vi "test.vi"() -> ()   [LabVIEW 2010, in "FPGAWrapperAK101022Resonance.lvclass"]
uses:
  FPGAWrapperAK101022Resonance.lvclass
  scan_specification_cluster.ctl
  class_data.vi
  Program Files (x86)/National Instruments/LabVIEW 2010/resource/objmgr/ni.dex.rc
panel:
  in  "sine mode?":bool
  out "Intensity output":i16[](graph)
  in  "Intensity amplitude":dbl
  out "channelA 2D":dbl[][](graph)
  out "channelA":dbl[](array[numeric])
  out "Available Elements for Reading":i32
  out "DAQ loop error out":errorcluster
  out "FPGA_AK101022Resonance out":refnum<class "FPGAWrapperAK101022Resonance.lvclass">
  in  "scan specification":T1
  in  "number of channels":i32=2
  in  "block size":i32=10000
  out "channel data block":dbl[][](graph)
  in  "timeout (ms)":i32=500
  out "timed out?":bool
  out "DAQ loop counter":i32=9010145
  in  "run button":bool
  in  "stop":bool
  # "Test VI for FGPA_AK101022Resonance"
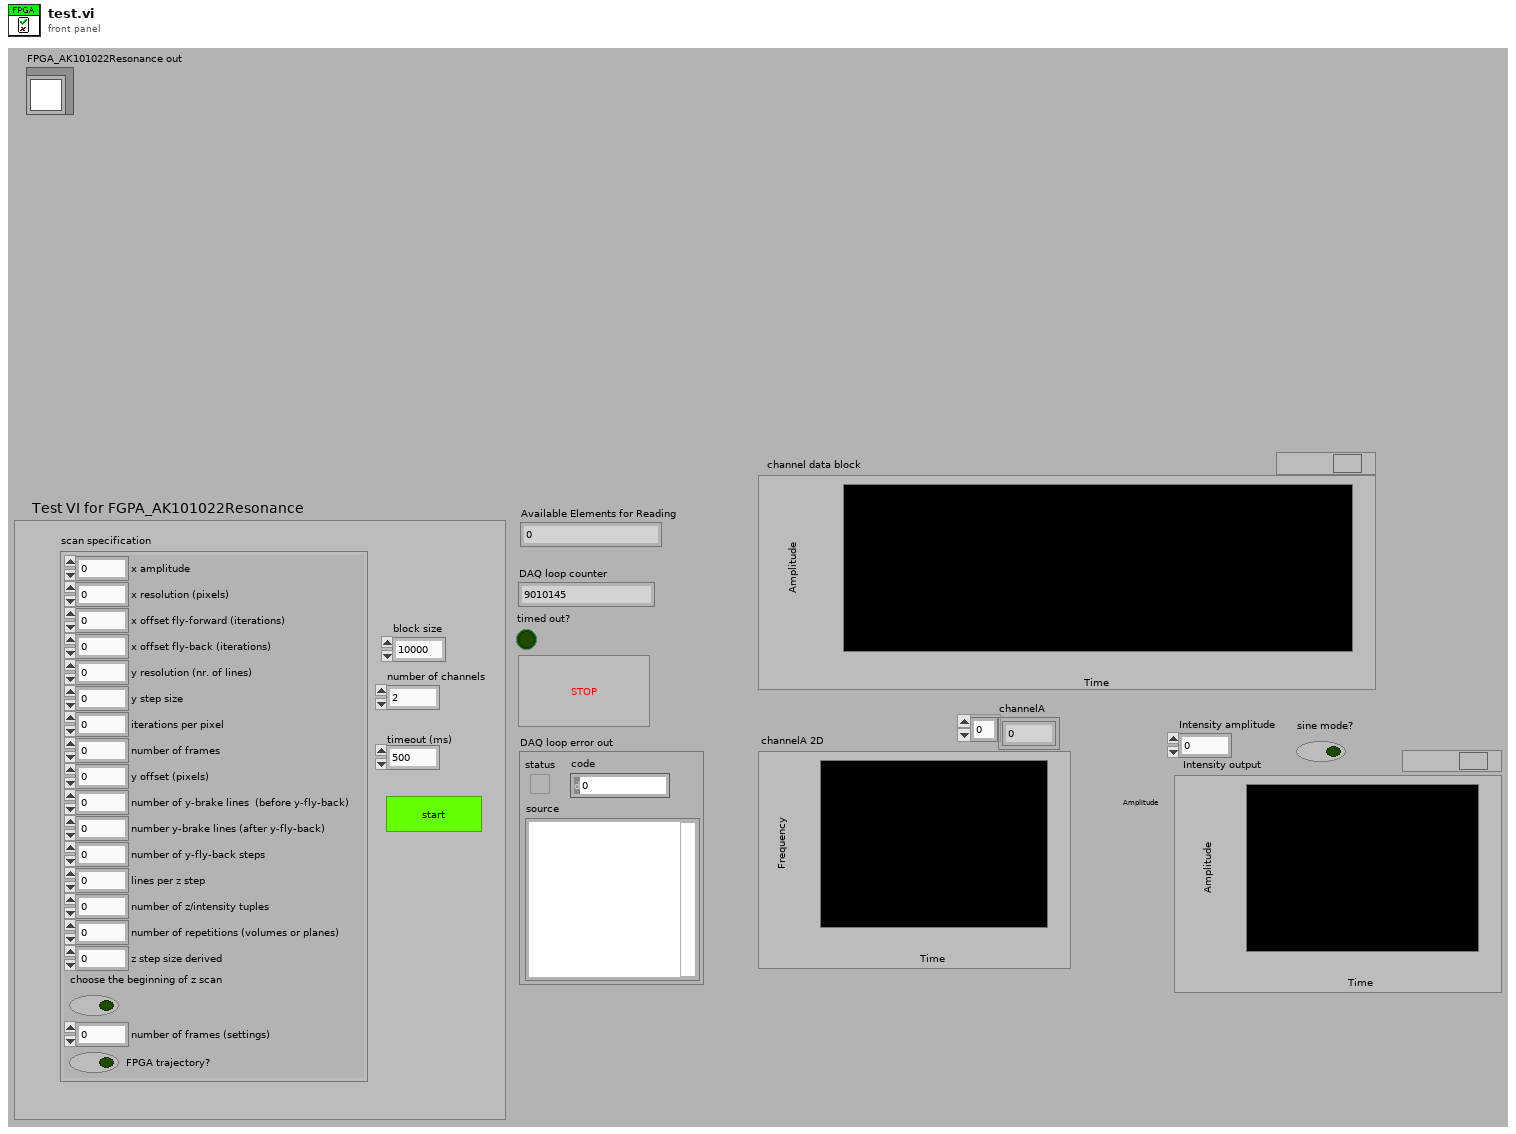
[diagram p1: front panel]
types:
  T1 = typedef "scan_specification_cluster.ctl" = cluster{"x amplitude":u16, "x resolution (pixels)":u16, "x offset fly-forward (iterations)":u16, "x offset fly-back (iterations)":u16, "y resolution (nr. of lines)":u16, "y step size":u16, "iterations per pixel":u16, "number of frames":i32, "y offset (pixels)":u16, "number of y-brake lines  (before y-fly-back)":u16, "number y-brake lines (after y-fly-back)":u16, "number of y-fly-back steps":u16, "lines per z step":u16, "number of z/intensity tuples":u16, "number of repetitions (volumes or planes)":i32, "z step size derived":u16, "choose the beginning of z scan":bool, "number of frames (settings)":i32, "FPGA trajectory?":bool}
  T2 = typedef "pixel_raw_data_array.ctl" = dbl[][]
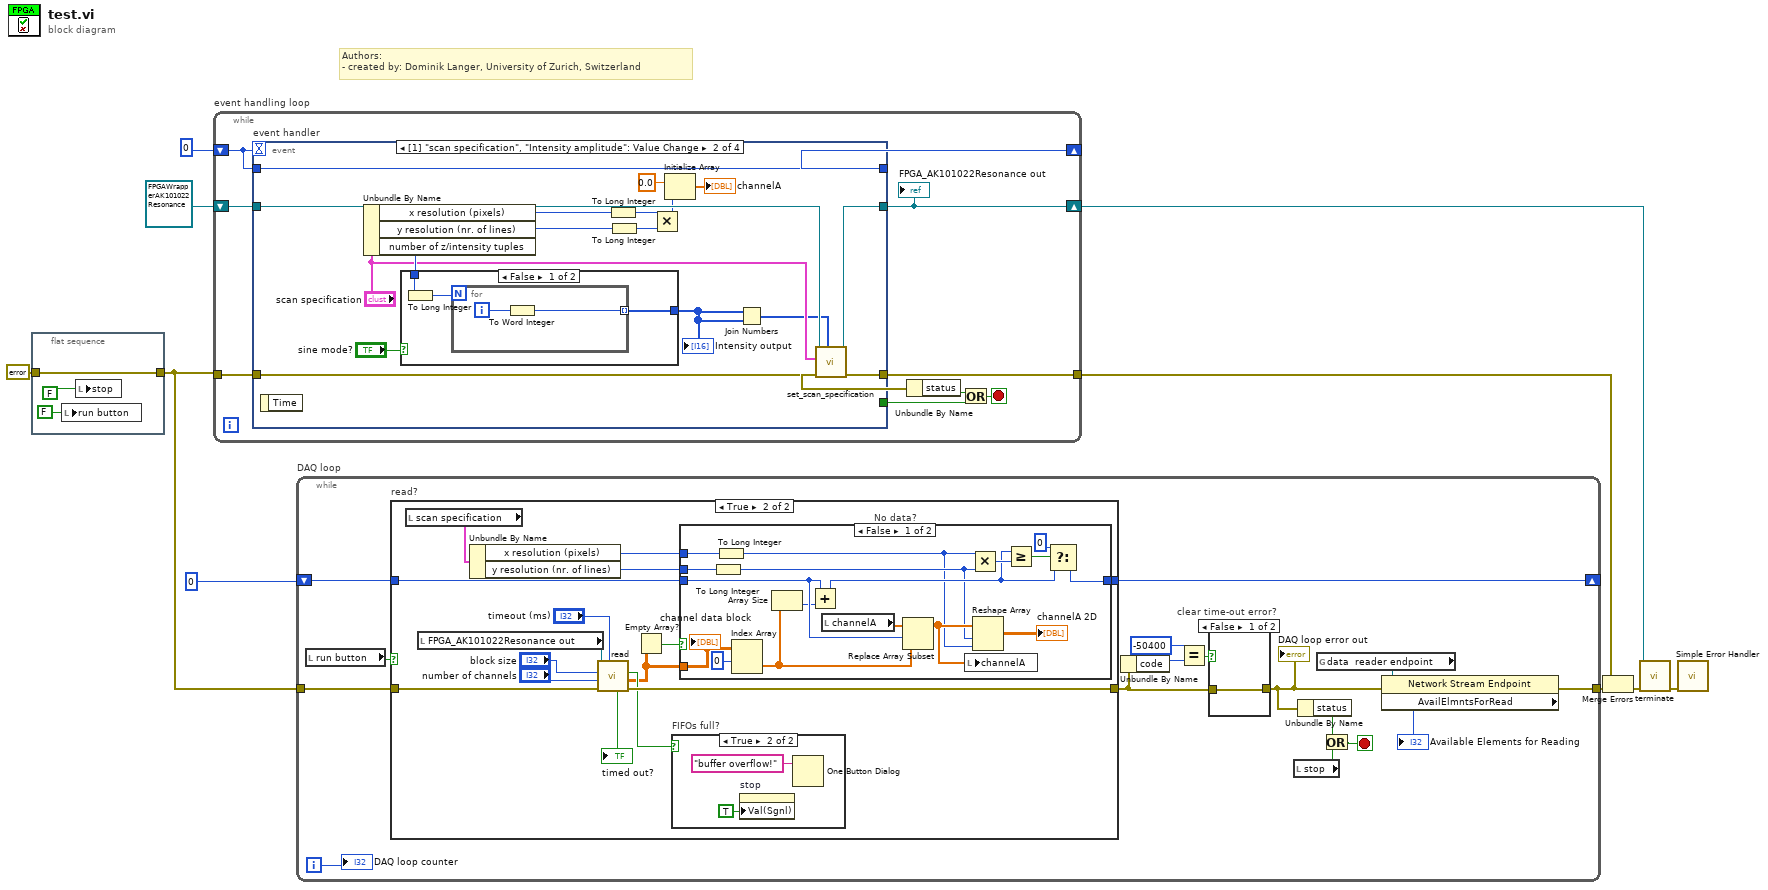
[diagram p0: block diagram]
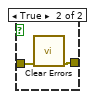
[diagram p2: hidden frame]
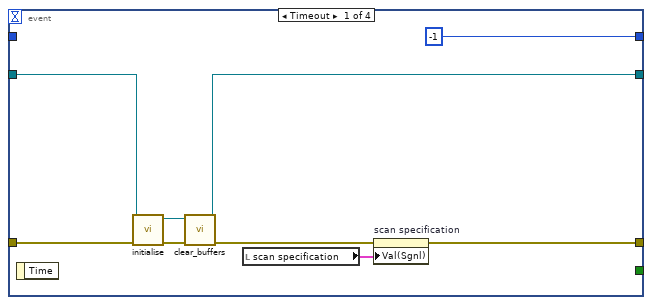
[diagram p6: hidden frame]
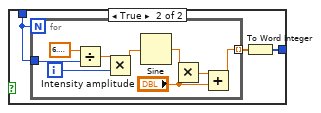
[diagram p7: hidden frame]
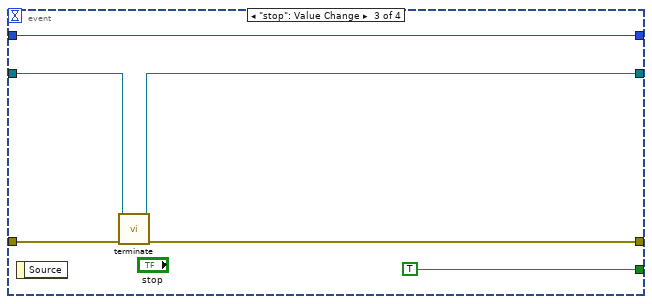
[diagram p8: hidden frame]
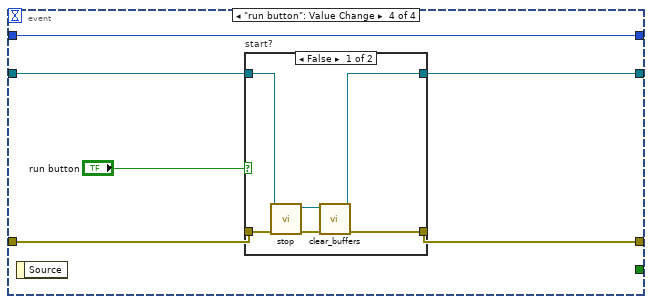
[diagram p9: hidden frame]
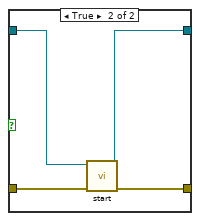
[diagram p10: hidden frame]
diagram:
  # "Authors: \n- created by: Dominik Langer, University of Zurich, Switzerland"
  n1 = flat-sequence {
    tunnel: errorcluster {"status"=FALSE, "code"=0, "source"=""} ("error in (no error)") -> [w13]
    tunnel: [w13] -> w2
    frame #0 {
      n2 = local write "run button"(FALSE ("run button")) -> ()
      n3 = local write "stop"(FALSE) -> ()
    }
  }
  n4 = while "event handling loop" {
    shift-right: [w20] -> _
    shift-left: 0 -> [w21]
    shift-right: [w18] -> w8
    shift-left: refnum<class "FPGAWrapperAK101022Resonance.lvclass"> refnum ("FPGA_AK101022Resonance.lvclass") -> [w19]
    tunnel: w2 -> [w22]
    tunnel: [w17] -> w7
    stop <- w14 stop-if-true
    n5 = event "event handler" shown="[1] \"scan specification\", \"Intensity amplitude\": Value Change" {
      selector: _ -> [_ _ _ _]
      dyn-events: _ -> [_ _ _ _]
      timeout: w21 -> [_ _ _ _]
      tunnel: [w28 w44 w68 w72] -> w17
      tunnel: w22 -> [w29 w45 w69 w76]
      tunnel: w21 -> [_ w48 w71 w77]
      tunnel: [-1 w48 w71 w77] -> w20
      tunnel: [_ _ TRUE _] -> w15
      tunnel: [w24 w46 w66 w73] -> w18
      tunnel: w19 -> [w30 w47 w67 w74]
      event Timeout {
        n6 = event-data() -> ()  [unwired: 2 out]
        n7 = call-dynamic "initialise.vi"("error in (no error)"=w29, "FPGA_AK101022Resonance in"=w30) -> ("error out"=w27:errorcluster, "FPGA_AK101022Resonance out"=w25:refnum<class "FPGAWrapperAK101022Resonance.lvclass">)  [unwired: 8 in]
        n8 = call-dynamic "clear_buffers.vi"("error in (no error)"=w27, "FPGA_AK101022Resonance in"=w25) -> ("error out"=w26:errorcluster, "FPGA_AK101022Resonance out"=w24:refnum<class "FPGAWrapperAK101022Resonance.lvclass">)  [unwired: 8 in]
        n9 = local read "scan specification"() -> (w23:T1)
        n10 = property on="scan specification" class="Clust (strict)"(error in=w26, "Val(Sgnl)"=w23) -> (error out=w28:errorcluster)  [unwired: 1 in, 1 out]
      }
      event "Intensity amplitude": Value Change {
        n11 = event-data() -> ()  [unwired: 2 out]
        n12 = Unbundle By Name("scan specification") -> ("x resolution (pixels)"=w42:u16, "y resolution (nr. of lines)"=w38:u16, "number of z/intensity tuples"=w36:u16)
        n13 = case shown="False" "sine mode?" {
          tunnel: w36 -> [w50 w56]
          tunnel: [w51 w54] -> w33
          frame False {
            n14 = To Long Integer(number=w50) -> (32bit integer=w49:i32)
            n15 = for {
              N: w49 -> [_]
              tunnel: [w52] -> w51 mode=indexing
              i -> [w53]
              n16 = To Word Integer(number=w53) -> (16bit integer=w52:i16)
            }
          }
          frame True {
            n17 = for {
              N: w56 -> [_]
              tunnel: w56 -> [w64]
              tunnel: [w57] -> w55 mode=indexing
              i -> [w62]
              n18 = Divide(x=6.283185307179586, y=w64) -> (x/y=w63:dbl)
              n19 = Multiply(x=w63, y=w62) -> (x*y=w61:dbl)
              n20 = Sine(x=w61) -> (sin(x)=w60:dbl)
              n21 = Multiply(x=w60, y="Intensity amplitude") -> (x*y=w59:dbl)
              n22 = Add(x=w59, y="Intensity amplitude") -> (x+y=w57:dbl)
            }
            n23 = To Word Integer(number=w55) -> (16bit integer=w54:i16[])
          }
        }
        "Intensity output" <- w33
        n24 = To Long Integer(number=w42) -> (32bit integer=w39:i32)
        n25 = To Long Integer(number=w38) -> (32bit integer=w37:i32)
        n26 = Multiply(x=w39, y=w37) -> (x*y=w40:i32)
        n27 = Initialize Array(0.0 ("element"), w40) -> (→"channelA":dbl[])
        n28 = Join Numbers(hi=w33, lo=w33) -> ((hi.lo)=w32:u32[])
        n29 = call-dynamic "set_scan_specification.vi"("z/intensity tuples (U32: high U16 is z, low U16 is intensity)"=w32, "error in (no error)"=w45, "scan specification"="scan specification", "FPGA_AK101022Resonance in"=w47) -> ("error out"=w44:errorcluster, "FPGA_AK101022Resonance out"=w46:refnum<class "FPGAWrapperAK101022Resonance.lvclass">)  [unwired: 6 in]
      }
      event "stop": Value Change {
        n30 = event-data() -> ()  [unwired: 2 out]
        n31 = call-dynamic "terminate.vi"("error in (no error)"=w69, "FPGA_AK101022Resonance in"=w67) -> ("error out"=w68:errorcluster, "FPGA_AK101022Resonance out"=w66:refnum<class "FPGAWrapperAK101022Resonance.lvclass">)  [unwired: 8 in]
      }
      event "run button": Value Change {
        n32 = event-data() -> ()  [unwired: 2 out]
        n33 = case "start?" shown="False" "run button" {
          tunnel: w76 -> [w83 w85]
          tunnel: w74 -> [w82 w84]
          tunnel: [w78 w87] -> w73
          tunnel: [w80 w86] -> w72
          frame False {
            n34 = call-dynamic "stop.vi"("error in (no error)"=w83, "FPGA_AK101022Resonance in"=w82) -> ("error out"=w81:errorcluster, "FPGA_AK101022Resonance out"=w79:refnum<class "FPGAWrapperAK101022Resonance.lvclass">)  [unwired: 8 out]
            n35 = call-dynamic "clear_buffers.vi"("error in (no error)"=w81, "FPGA_AK101022Resonance in"=w79) -> ("error out"=w80:errorcluster, "FPGA_AK101022Resonance out"=w78:refnum<class "FPGAWrapperAK101022Resonance.lvclass">)  [unwired: 8 in]
          }
          frame True {
            n36 = call-dynamic "start.vi"("error in (no error)"=w85, "FPGA_AK101022Resonance in"=w84) -> ("error out"=w86:errorcluster, "FPGA_AK101022Resonance out"=w87:refnum<class "FPGAWrapperAK101022Resonance.lvclass">)  [unwired: 8 out]
          }
        }
      }
    }
    "FPGA_AK101022Resonance out" <- w18
    n37 = Unbundle By Name(w17) -> ("status"=w16:bool)
    n38 = Or(x=w16, y=w15) -> (x .or. y?=w14:bool)
  }
  n39 = while "DAQ loop" {
    tunnel: w2 -> [w103]
    tunnel: [w91] -> w9
    shift-right: [w88] -> _
    shift-left: 0 -> [w89]
    i -> [w94]
    stop <- w95 stop-if-true
    n40 = local read "run button"() -> (w102:bool)
    n41 = case "read?" shown="True" w102 {
      tunnel: w103 -> [w107 w122]
      tunnel: [w107 w121] -> w99
      tunnel: w89 -> [_ w112]
      tunnel: [_ w111] -> w88
      frame False {
      }
      frame True {
        n42 = local read "scan specification"() -> (w110:T1)
        n43 = local read "FPGA_AK101022Resonance out"() -> (w115:refnum<class "FPGAWrapperAK101022Resonance.lvclass">)
        n44 = Unbundle By Name(w110) -> ("x resolution (pixels)"=w108:u16, "y resolution (nr. of lines)"=w109:u16)
        n45 = call-dynamic "read.vi"("timeout (ms)"="timeout (ms)", "error in (no error)"=w122, "number of channels"="number of channels", "block size"="block size", "FPGA_AK101022Resonance in"=w115) -> ("error out"=w121:errorcluster, "channels raw data block"=w113:T2, "FIFO full?"=w118:bool, "timed out?"=→"timed out?":bool)  [unwired: 3 out]
        n46 = Empty Array?(array=w113) -> (empty?=w114:bool)
        n47 = case "FIFOs full?" shown="True" w118 {
          frame False {
          }
          frame True {
            n48 = property on="stop" class="Bool (strict)"("Val(Sgnl)"=TRUE) -> ()  [unwired: 2 in, 2 out]
            n49 = One Button Dialog(message="buffer overflow!") -> ()  [unwired: 1 in, 1 out]
          }
        }
        n50 = case "No data?" shown="False" w114 {
          tunnel: w113 -> [w141 _]
          tunnel: w112 -> [w139 w142]
          tunnel: [w132 w142] -> w111
          tunnel: w108 -> [w137 _]
          tunnel: w109 -> [w136 _]
          frame False {
            n51 = To Long Integer(number=w136) -> (32bit integer=w128:i32)
            n52 = To Long Integer(number=w137) -> (32bit integer=w127:i32)
            n53 = Index Array(array=w141, index (row)=0) -> (element=w126:dbl[])  [unwired: 1 in]
            n54 = Array Size(array=w126) -> (size(s)=w125:i32)
            n55 = Add(x=w139, y=w125) -> (x+y=w133:i32)
            n56 = local read "channelA"() -> (w140:dbl[])
            n57 = Replace Array Subset(array=w140, new element=w126, index=w139) -> (w129:dbl[])
            n58 = local write "channelA"(w129) -> ()
            n59 = Multiply(x=w127, y=w128) -> (x*y=w135:i32)
            n60 = Reshape Array(w129, w128, w127) -> (→"channelA 2D":dbl[][])
            n61 = Greater Or Equal?(x=w133, y=w135) -> (x >= y?=w134:bool)
            n62 = Select(t=0, s=w134, f=w133) -> (s? t:f=w132:i32)
            "channel data block" <- w141
          }
          frame True {
          }
        }
      }
    }
    n63 = Unbundle By Name(w99) -> ("code"=w101:i32)
    n64 = Equal?(x=-50400, y=w101) -> (x = y?=w98:bool)
    n65 = case "clear time-out error?" shown="False" w98 {
      tunnel: w99 -> [w104 w106]
      tunnel: [w104 w105] -> w92
      frame False {
      }
      frame True {
        n66 = call <vilib>:"Clear Errors.vi"("error in (no error)"=w106) -> ("error out"=w105:errorcluster)  [unwired: 6 out]
      }
    }
    "DAQ loop error out" <- w92
    n67 = local read "stop"() -> (w96:bool)
    n68 = Unbundle By Name(w92) -> ("status"=w97:bool)
    n69 = global read "class_data.vi" "data  reader endpoint"() -> (w93:refnum<k21>)
    n70 = Or(x=w97, y=w96) -> (x .or. y?=w95:bool)
    n71 = property class="Network Stream Endpoint"(reference=w93, error in=w92) -> (error out=w91:errorcluster, "AvailElmntsForRead"=→"Available Elements for Reading":i32)  [unwired: 1 out]
    "DAQ loop counter" <- w94
  }
  n72 = call-dynamic "terminate.vi"("error in (no error)"=w9, "FPGA_AK101022Resonance in"=w8) -> ("error out"=w6:errorcluster)  [unwired: 9 out]
  n73 = Merge Errors(w7, w6) -> (w5:errorcluster)
  n74 = call <vilib>:"Simple Error Handler.vi"("error in (no error)"=w5) -> ()  [unwired: 1 in, 8 out]
